vi "Error - Fire Error.vi"(8 "error in (no error)":errorcluster, 9 "Error Data":variant, 10 "Error Type":T1, 11 "View Model":T2) -> (0 "error out":errorcluster, 3 "View Model":T2)   [LabVIEW 2017]
uses:
  Model/Controls/View Model.ctl
  Model/Controls/Shared Model.ctl
  Controls/Error Model.ctl
  Controls/Error Message.ctl
  Controls/Error Type.ctl
  Configuration/Controls/Config Model.ctl
  Configuration/Controls/Config DB Message.ctl
  Configuration/Controls/Config DB Command.ctl
  Configuration/Controls/Config DB Overhead.ctl
  Configuration/Controls/Config DB Record1.ctl
  Configuration/Controls/Config DB Record2.ctl
  Controller/Controls/Controller Wash Step.ctl
  Views/Vehicle Position Simulation View/Controls/Vehicle - Position.ctl
  Controller/Controls/Controller Model.ctl
  Controller/Controls/Controller Overhead.ctl
  Controller/Controls/Controller State.ctl
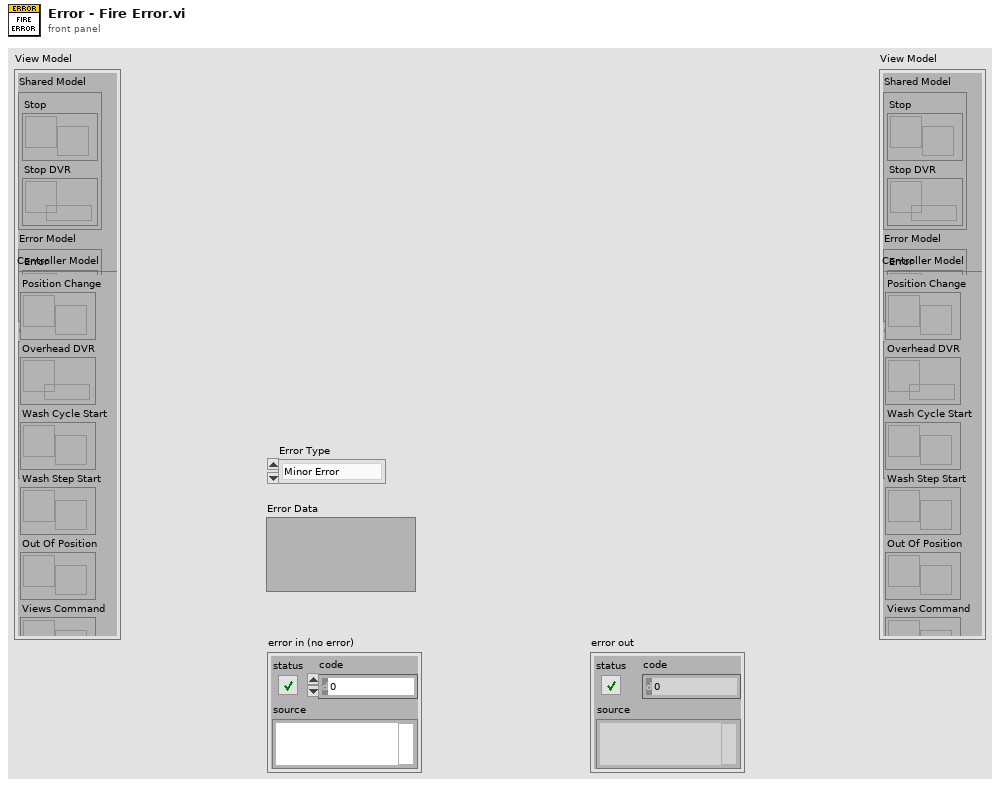
[diagram p1: front panel]
types:
  T1 = typedef "Error Type.ctl" = enum16{"Minor Error", "Wash Cycle Error", "System Error", "Unknown"}
  T2 = typedef "View Model.ctl" = cluster{"Shared Model":T3, "Error Model":T4, "Config Model":T5, "Controller Model":T6}
  T3 = typedef "Shared Model.ctl" = cluster{"Stop":refnum<user-event>, "Stop DVR":refnum<data-value>}
  T4 = typedef "Error Model.ctl" = cluster{"Error":refnum<user-event>}
  T5 = typedef "Config Model.ctl" = cluster{"Config":refnum<user-event>, "Config DVR":refnum<data-value>}
  T6 = typedef "Controller Model.ctl" = cluster{"Position Change":refnum<user-event>, "Overhead DVR":refnum<data-value>, "Wash Cycle Start":refnum<user-event>, "Wash Step Start":refnum<user-event>, "Out Of Position":refnum<user-event>, "Views Command":refnum<user-event>}
  T7 = typedef "Error Message.ctl" = cluster{"Error Type":T1, "Error Data":variant}
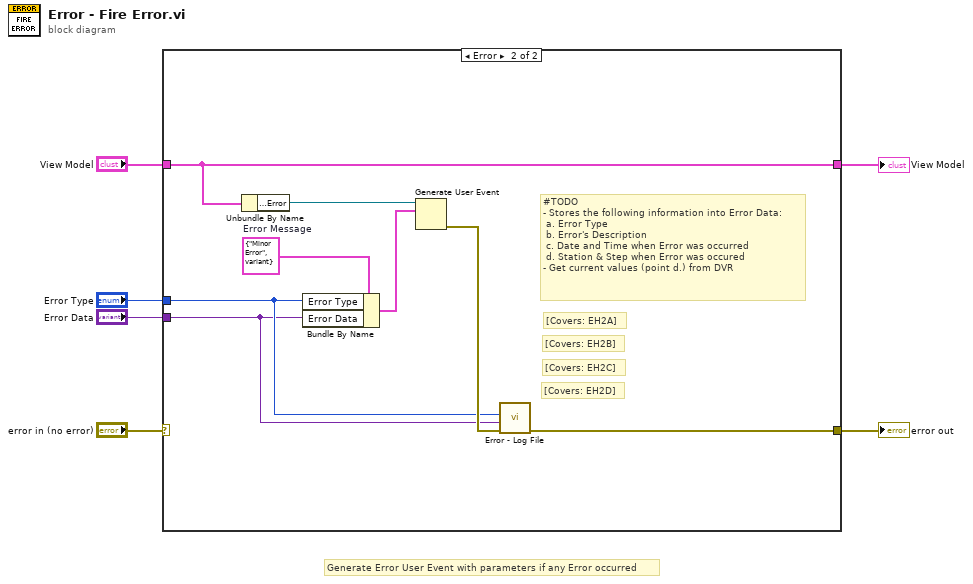
[diagram p0: block diagram]
diagram:
  # "Generate Error User Event with parameters if any Error occurred"
  n1 = case shown="Error" "error in (no error)" {
    selector: "error in (no error)" -> [w8 _]
    tunnel: "View Model" -> [w7 w9]
    tunnel: [w8 w12] -> w4
    tunnel: [w7 w9] -> w3
    tunnel: "Error Data" -> [_ w10]
    tunnel: "Error Type" -> [_ w11]
    frame No Error {
    }
    frame Error {
      w15 = T7 {"Error Type"=enum."Minor Error", "Error Data"=variant}  # Error Message
      # "[Covers: EH2D]"
      # "[Covers: EH2C]"
      # "[Covers: EH2B]"
      # "[Covers: EH2A]"
      # "#TODO\n- Stores the following information into Error Data:\n a. Error Type\n b. Error's Description\n c. Date and Time when Error was occurred\n d. Station & Step when Error was occured\n- Get current values (point d.) from DVR"
      n2 = Unbundle By Name(w9) -> ("Error Model.Error"=w16:refnum<user-event>)
      n3 = Bundle By Name(cluster=w15, "Error Type"=w11, "Error Data"=w10) -> (w14:T7)
      n4 = Generate User Event(user event=w16, event data cluster=w14) -> (error out=w13:errorcluster)  [unwired: 2 in, 1 out]
      n5 = call "Error - Log File.vi"("error in (no error)"=w13, "Error Data"=w10, "Error Type"=w11) -> ("error out"=w12:errorcluster)  [unwired: 8 in]
    }
  }
  "View Model" <- w3
  "error out" <- w4
